vi "FlattenStrPtr To MDPtr.vi"(1 "FlattenStrPtr":string) -> (0 "HexStrPtr":T1)   [LabVIEW 2017]
uses:
  MDPtr TypeDef/MDPtr.ctl
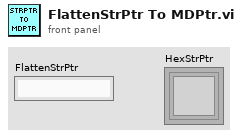
[diagram p1: front panel]
types:
  T1 = typedef "MDPtr.ctl" = refnum<k1>
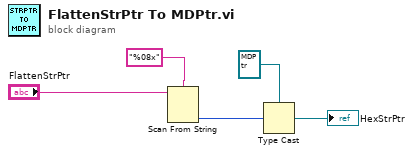
[diagram p0: block diagram]
diagram:
  n1 = Scan From String(format string="%08x", input string="FlattenStrPtr") -> (output 1=w2:u32)  [unwired: 3 in, 3 out]
  n2 = Type Cast(type=T1 refnum ("MDPtr"), x=w2) -> (*(type *) &x=→"HexStrPtr":T1)
